vi "get Flash FileName .vi"(6 "Light Correction":string, 7 "Time":timestamp, 8 "Device Name":string, 9 "Operator":string="Radek", 10 "Wafer Name":string, 11 "FineTest save path":path=path "C:/Users/Flash/Desktop/Data/Detector test data/IV") -> (3 "appended path":path)   [LabVIEW 2012]
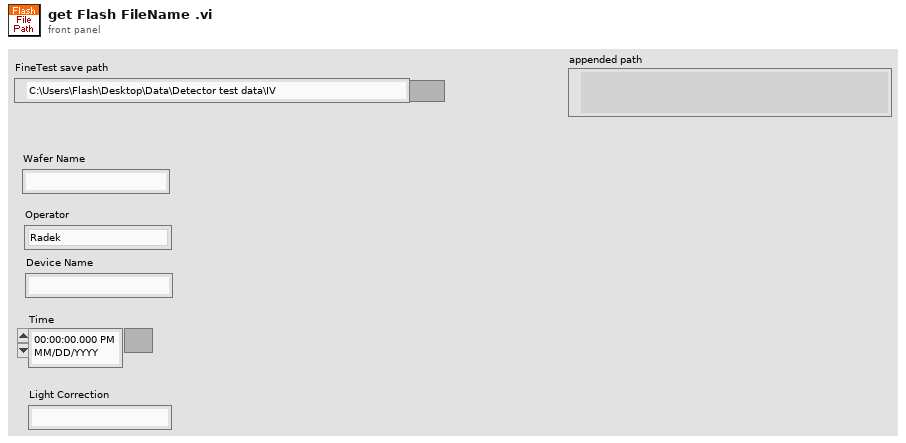
[diagram p1: front panel]
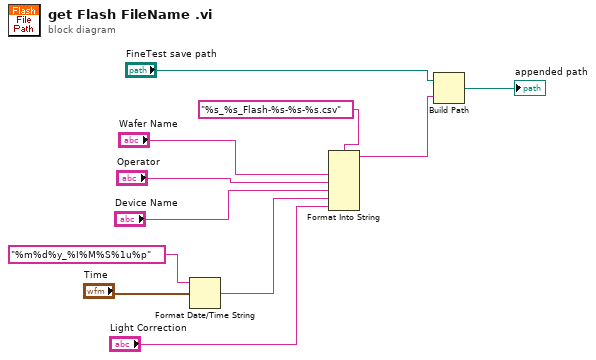
[diagram p0: block diagram]
diagram:
  n1 = Format Date/Time String(time format string (%c)="%m%d%y_%I%M%S%1u%p", seconds (now)="Time") -> (date/time string=w6:string)  [unwired: 1 in]
  n2 = Format Into String(format string="%s_%s_Flash-%s-%s-%s.csv", "Wafer Name", "Operator", "Device Name", w6, "Light Correction") -> (resulting string=w2:string)  [unwired: 2 in, 1 out]
  n3 = Build Path(base path="FineTest save path", name or relative path=w2) -> (appended path=→"appended path":path)
